vi "Calculate Function.vi"(0 "Instrument Handle In":i32, 1 "Source2":i32(ring) caption="Source 2" items=["Input Channel 1", "Input Channel 2", "Input Channel 3", "Input Channel 4", "Calc Channel 1", "Calc Channel 2", "Calc Channel 3", "Calc Channel 4", "Ref Channel 1", "Ref Channel 2", "Ref Channel 3", "Ref Channel 4"], 2 "Range Offset Mode":i32(ring) caption="Range & Offset Mode" items=["Auto", "Manual"], 5 "Calculation Channel":i32(ring) items=["Calc Channel 1", "Calc Channel 2", "Calc Channel 3", "Calc Channel 4"], 7 "Source1":i32(ring) caption="Source 1" items=["Input Channel 1", "Input Channel 2", "Input Channel 3", "Input Channel 4", "Calc Channel 1", "Calc Channel 2", "Calc Channel 3", "Calc Channel 4", "Ref Channel  1", "Ref Channel 2", "Ref Channel 3", "Ref Channel 4"], 9 "Operation":i32(ring) items=["Add", "Absolute Value", "Copy", "Derivative", "Integral", "Inverse", "Multiply", "Subtract", "Limit Test", "FFT", "Smooth", "Measurement", "Histogram", "No Operation"], 11 "error in":errorcluster, 12 "Range":dbl, 13 "Offset":dbl) -> (4 "Instrument Handle Out":i32, 15 "error out":errorcluster)   [LabVIEW 8.6, in "ZTScopeM.lvlib"]
doc: "Set a calculation channel to perform an operation and configure basic channel settings."
uses:
  ZTScopeM.lvlib
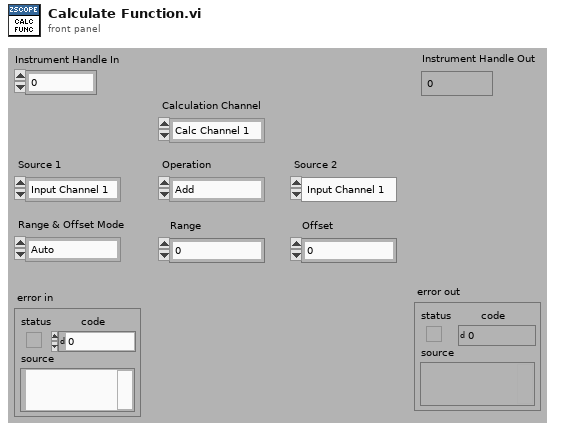
[diagram p1: front panel]
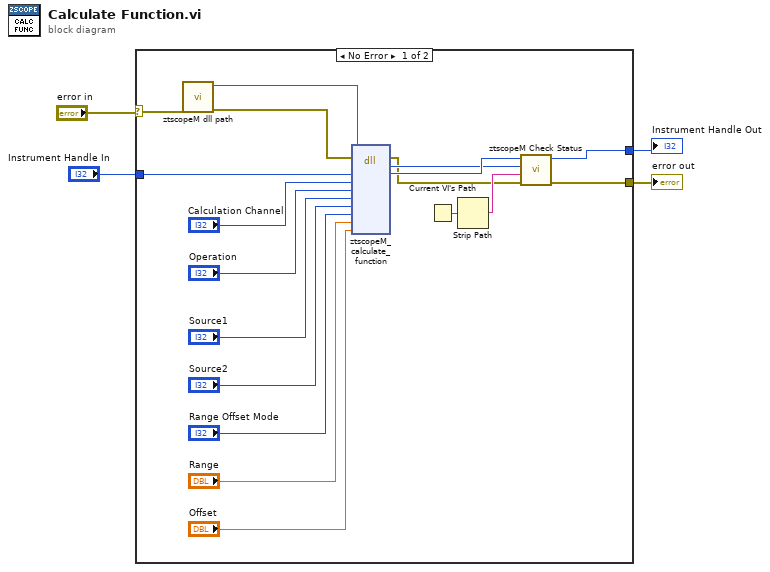
[diagram p0: block diagram]
diagram:
  n1 = case shown="No Error" "error in" {
    selector: "error in" -> [w8 w24]
    tunnel: [w10 w24] -> w1
    tunnel: "Instrument Handle In" -> [w22 w23]
    tunnel: [w9 w23] -> w3
    frame #0 {
      n2 = call "ztscopeM dll path.vi"("error in (no error)"=w8) -> ("error out"=w6:errorcluster, "<instrument>.dll path"=w7:path)  [unwired: 9 in]
      n3 = dll-call lib="C:/Program Files (x86)/National Instruments/LabVIEW 2013/instr.lib/ztscopem/ztscopeM.dll" fn="ztscopeM_calculate_function"(path in=w7, error in=w6, "instrumentHandle"=w22, "calculationChannel"="Calculation Channel", "operation"="Operation", "source1"="Source1", "source2"="Source2", "rangeOffsetMode"="Range Offset Mode", "range"="Range", "offset"="Offset") -> (error out=w5:errorcluster, w11:i32, "instrumentHandle"=w12:i32)  [unwired: 8 in, 1 out]
      n4 = Current VI's Path() -> (path=w14:path)
      n5 = Strip Path(path=w14) -> (name=w13:string)  [unwired: 1 out]
      n6 = call "ztscopeM Check Status.vi"("error in"=w5, "name of VI"=w13, "status (return code)"=w11, "instrument handle in"=w12) -> ("error out"=w10:errorcluster, "instrument handle out"=w9:i32)  [unwired: 2 in]
    }
    frame #1 {
    }
  }
  "Instrument Handle Out" <- w3
  "error out" <- w1
